vi "DriveEnc.vi"(11 "Reset?":bool) -> (0 "RightEncder":dbl, 3 "LeftEncoder":dbl)   [LabVIEW 2017]
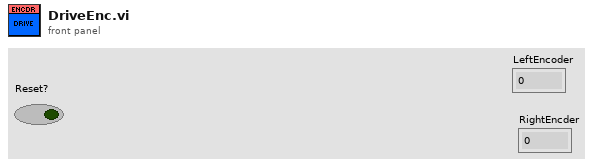
[diagram p1: front panel]
types:
  T1 = typedef "WPI_EncoderDevRef.ctl" = cluster{"DevStatus":errorcluster, "EncoderIndex":T2, "CounterIndex":T3, "DistancePerCount":dbl, "Decoding Type":T4}
  T2 = typedef "FPGA_EncoderIdx.ctl" = enum8{"Enc 0", "Enc 1", "Enc 2", "Enc 3", "Enc 4", "Enc 5", "Enc 6", "Enc 7", "Invalid"}
  T3 = typedef "FPGA_CounterCtrSystemIndex.ctl" = enum8{"Ctr 0", "Ctr 1", "Ctr 2", "Ctr 3", "Ctr 4", "Ctr 5", "Ctr 6", "Ctr 7", "Invalid"}
  T4 = typedef "WPI_EncoderType.ctl" = enum16{"1x", "2x", "4x"}
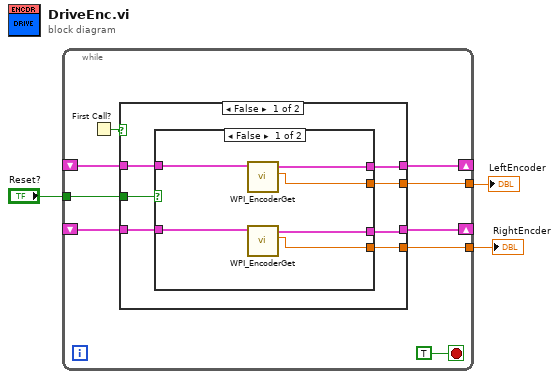
[diagram p0: block diagram]
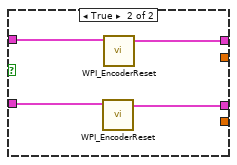
[diagram p2: hidden frame]
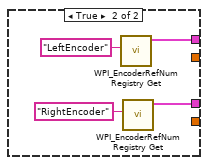
[diagram p3: hidden frame]
diagram:
  n1 = while {
    shift-right: [w9] -> _
    shift-left: _ -> [w7]
    shift-right: [w10] -> _
    shift-left: _ -> [w8]
    tunnel: "Reset?" -> [w6]
    tunnel: [w5] -> w2
    tunnel: [w4] -> w1
    stop <- TRUE stop-if-true
    n2 = First Call?() -> (First Call?: T/F=w12:bool)
    n3 = case shown="False" w12 {
      tunnel: [w15 w31] -> w10
      tunnel: [w16 w30] -> w9
      tunnel: w8 -> [w17 _]
      tunnel: w7 -> [w18 _]
      tunnel: w6 -> [w19 _]
      tunnel: [w14 _] -> w5
      tunnel: [w13 _] -> w4
      frame False {
        n4 = case shown="False" w19 {
          tunnel: w18 -> [w25 w29]
          tunnel: w17 -> [w22 w27]
          tunnel: [w24 w28] -> w16
          tunnel: [w23 w26] -> w15
          tunnel: [w21 _] -> w14
          tunnel: [w20 _] -> w13
          frame False {
            n5 = call <vilib>:"WPI_EncoderGet.vi"("EncoderDevRef"=w25) -> ("Distance"=w21:dbl, "EncoderDevRef"=w24:T1)  [unwired: 5 in, 4 out]
            n6 = call <vilib>:"WPI_EncoderGet.vi"("EncoderDevRef"=w22) -> ("Distance"=w20:dbl, "EncoderDevRef"=w23:T1)  [unwired: 5 in, 4 out]
          }
          frame True {
            n7 = call <vilib>:"WPI_EncoderReset.vi"("EncoderDevRef"=w27) -> ("EncoderDevRef"=w26:T1)  [unwired: 9 in, 1 out]
            n8 = call <vilib>:"WPI_EncoderReset.vi"("EncoderDevRef"=w29) -> ("EncoderDevRef"=w28:T1)  [unwired: 9 in, 1 out]
          }
        }
      }
      frame True {
        n9 = call <vilib>:"WPI_EncoderRefNum Registry Get.vi"("refnum name"="LeftEncoder") -> ("EncoderDevRef"=w30:T1)  [unwired: 9 in, 1 out]
        n10 = call <vilib>:"WPI_EncoderRefNum Registry Get.vi"("refnum name"="RightEncoder") -> ("EncoderDevRef"=w31:T1)  [unwired: 9 in, 1 out]
      }
    }
  }
  "LeftEncoder" <- w2
  "RightEncder" <- w1
